vi "Init cDAQ.vi"(8 "error in":errorcluster, 11 "Data in":T1={"Config"={"Hipot"={"COM PORT"=0, "AC to Pack"={"Mode"=0, "Voltage Level"=1000.0, "Low Limit"=0.0, "Hi Limit"=0.001, "ARC Limit"=0.0, "Step"=1.0, "Ramp Time "=0.0, "Test Time "=3.0}, "AC to Pack IR"={"Mode"=0, "Voltage Level IR"=1000.0, "Low Limit"=10000000.0, "Hi Limit"=0.001, "Real Current Limit"=0.0, "Step"=1.0, "Ramp Time "=0.0, "Test Time "=3.0}, "Pack to Case"={"Mode"=0, "Voltage Level"=1000.0, "Low Limit"=10000000.0, "Hi Limit"=0.0, "ARC Limit"=1.0, "Step"=0.0, "Ramp Time "=3.0, "Test Time "=3.0}, "Pack to Case IR"={"Mode"=0, "Voltage Level IR"=1000.0, "Low Limit"=10000000.0, "Hi Limit"=0.0, "Real Current Limit"=0.0, "Step"=1.0, "Ramp Time "=0.0, "Test Time "=3.0}}, "62150H-600 Supply"={"IVI Resource Name"=""}, "6320X E Load Heater"={"IVI Resource Name"=""}, "6320X E Load Compressor"={"IVI Resource Name"=""}, "6320X E Load DCDC"={"IVI Resource Name"=""}, "12061 DMM"={"IVI Resource Name"=""}, "17040 Pack Regen"={"IVI Resource Name"=""}}, "Test Data Ref"=refnum, "Current State Ref"=refnum, "Hipot Ref"=refnum, "Contactors Ref"=refnum, "Equipment Status Ref"=refnum, "TX Packet Info Ref"=refnum, "Pcap Cluster Ref"=refnum, "Eth Adapter ID Ref"=refnum, "Pass/Fail Results Ref"=refnum, "Sequence to Send Ref"=refnum, "Transmit Btn Ref"=refnum, "HW Handles Ref"=refnum, "MPB Status Ref"=refnum, "HVIL Source Ref"=refnum, "HVIL Readback Ref"=refnum, "Coolant Flow Ref"=refnum, "Coolant Temp Ref"=refnum, "Chiller Valve Open % Ref"=refnum} {"Config"."Hipot"."Pack to Case IR"."Test Time" min=0.0 max=999.0 step=0.1 format="%.1f"; "Config"."Hipot"."Pack to Case IR"."Ramp Time" min=0.0 max=999.0 step=0.1 format="%.1f"; "Config"."Hipot"."Pack to Case IR"."Step" min=1.0 max=99.0 step=1.0; "Config"."Hipot"."Pack to Case IR"."Real Current Limit" min=0.0 max=0.03 step=1e-06 format="%.2p"; "Config"."Hipot"."Pack to Case IR"."Voltage Level IR" min=100.0 max=1000.0 step=2.0; "Config"."Hipot"."Pack to Case IR"."Hi Limit" min=0.0 max=50000000000.0 step=10000.0 format="%.2p"; "Config"."Hipot"."Pack to Case IR"."Low Limit" min=100000.0 max=50000000000.0 step=10000.0 format="%.2p"; "Config"."Hipot"."Pack to Case IR"."Mode" items=["AC", "DC", "IR"]; "Config"."Hipot"."Pack to Case"."Test Time" min=0.0 max=999.0 step=0.1 format="%.1f"; "Config"."Hipot"."Pack to Case"."Ramp Time" min=0.0 max=999.0 step=0.1 format="%.1f"; "Config"."Hipot"."Pack to Case"."Step" min=1.0 max=99.0 step=1.0; "Config"."Hipot"."Pack to Case"."ARC Limit" min=0.0 max=0.015 step=1e-06 format="%.2p"; "Config"."Hipot"."Pack to Case"."Hi Limit" min=1e-06 max=0.03 step=1e-06 format="%.2p"; "Config"."Hipot"."Pack to Case"."Low Limit" min=0.0 max=0.03 step=1e-06 format="%.2p"; "Config"."Hipot"."Pack to Case"."Voltage Level" min=100.0 max=6000.0 step=2.0; "Config"."Hipot"."Pack to Case"."Mode" items=["AC", "DC", "IR"]; "Config"."Hipot"."AC to Pack IR"."Test Time" min=0.0 max=999.0 step=0.1 format="%.1f"; "Config"."Hipot"."AC to Pack IR"."Ramp Time" min=0.0 max=999.0 step=0.1 format="%.1f"; "Config"."Hipot"."AC to Pack IR"."Step" min=1.0 max=99.0 step=1.0; "Config"."Hipot"."AC to Pack IR"."Real Current Limit" min=0.0 max=0.03 step=1e-06 format="%.2p"; "Config"."Hipot"."AC to Pack IR"."Voltage Level IR" min=100.0 max=1000.0 step=2.0; "Config"."Hipot"."AC to Pack IR"."Hi Limit" min=0.0 max=50000000000.0 step=10000.0 format="%.2p"; "Config"."Hipot"."AC to Pack IR"."Low Limit" min=100000.0 max=50000000000.0 step=10000.0 format="%.2p"; "Config"."Hipot"."AC to Pack IR"."Mode" items=["AC", "DC", "IR"]; "Config"."Hipot"."AC to Pack"."Test Time" min=0.0 max=999.0 step=0.1 format="%.1f"; "Config"."Hipot"."AC to Pack"."Ramp Time" min=0.0 max=999.0 step=0.1 format="%.1f"; "Config"."Hipot"."AC to Pack"."Step" min=1.0 max=99.0 step=1.0; "Config"."Hipot"."AC to Pack"."ARC Limit" min=0.0 max=0.015 step=1e-06 format="%.2p"; "Config"."Hipot"."AC to Pack"."Hi Limit" min=1e-06 max=0.03 step=1e-06 format="%.2p"; "Config"."Hipot"."AC to Pack"."Low Limit" min=0.0 max=0.03 step=1e-06 format="%.2p"; "Config"."Hipot"."AC to Pack"."Voltage Level" min=100.0 max=6000.0 step=2.0; "Config"."Hipot"."AC to Pack"."Mode" items=["AC", "DC", "IR"]}) -> (0 "error out":errorcluster, 2 "Init cDAQ OK":bool, 3 "Data Out":T1={"Config"={"Hipot"={"COM PORT"=0, "AC to Pack"={"Mode"=0, "Voltage Level"=1000.0, "Low Limit"=0.0, "Hi Limit"=0.001, "ARC Limit"=0.0, "Step"=1.0, "Ramp Time "=0.0, "Test Time "=3.0}, "AC to Pack IR"={"Mode"=0, "Voltage Level IR"=1000.0, "Low Limit"=10000000.0, "Hi Limit"=0.001, "Real Current Limit"=0.0, "Step"=1.0, "Ramp Time "=0.0, "Test Time "=3.0}, "Pack to Case"={"Mode"=0, "Voltage Level"=1000.0, "Low Limit"=10000000.0, "Hi Limit"=0.0, "ARC Limit"=1.0, "Step"=0.0, "Ramp Time "=3.0, "Test Time "=3.0}, "Pack to Case IR"={"Mode"=0, "Voltage Level IR"=1000.0, "Low Limit"=10000000.0, "Hi Limit"=0.0, "Real Current Limit"=0.0, "Step"=1.0, "Ramp Time "=0.0, "Test Time "=3.0}}, "62150H-600 Supply"={"IVI Resource Name"=""}, "6320X E Load Heater"={"IVI Resource Name"=""}, "6320X E Load Compressor"={"IVI Resource Name"=""}, "6320X E Load DCDC"={"IVI Resource Name"=""}, "12061 DMM"={"IVI Resource Name"=""}, "17040 Pack Regen"={"IVI Resource Name"=""}}, "Test Data Ref"=refnum, "Current State Ref"=refnum, "Hipot Ref"=refnum, "Contactors Ref"=refnum, "Equipment Status Ref"=refnum, "TX Packet Info Ref"=refnum, "Pcap Cluster Ref"=refnum, "Eth Adapter ID Ref"=refnum, "Pass/Fail Results Ref"=refnum, "Sequence to Send Ref"=refnum, "Transmit Btn Ref"=refnum, "HW Handles Ref"=refnum, "MPB Status Ref"=refnum, "HVIL Source Ref"=refnum, "HVIL Readback Ref"=refnum, "Coolant Flow Ref"=refnum, "Coolant Temp Ref"=refnum, "Chiller Valve Open % Ref"=refnum} {"Config"."Hipot"."Pack to Case IR"."Test Time" min=0.0 max=999.0 step=0.1 format="%.1f"; "Config"."Hipot"."Pack to Case IR"."Ramp Time" min=0.0 max=999.0 step=0.1 format="%.1f"; "Config"."Hipot"."Pack to Case IR"."Step" min=1.0 max=99.0 step=1.0; "Config"."Hipot"."Pack to Case IR"."Real Current Limit" min=0.0 max=0.03 step=1e-06 format="%.2p"; "Config"."Hipot"."Pack to Case IR"."Voltage Level IR" min=100.0 max=1000.0 step=2.0; "Config"."Hipot"."Pack to Case IR"."Hi Limit" min=0.0 max=50000000000.0 step=10000.0 format="%.2p"; "Config"."Hipot"."Pack to Case IR"."Low Limit" min=100000.0 max=50000000000.0 step=10000.0 format="%.2p"; "Config"."Hipot"."Pack to Case IR"."Mode" items=["AC", "DC", "IR"]; "Config"."Hipot"."Pack to Case"."Test Time" min=0.0 max=999.0 step=0.1 format="%.1f"; "Config"."Hipot"."Pack to Case"."Ramp Time" min=0.0 max=999.0 step=0.1 format="%.1f"; "Config"."Hipot"."Pack to Case"."Step" min=1.0 max=99.0 step=1.0; "Config"."Hipot"."Pack to Case"."ARC Limit" min=0.0 max=0.015 step=1e-06 format="%.2p"; "Config"."Hipot"."Pack to Case"."Hi Limit" min=1e-06 max=0.03 step=1e-06 format="%.2p"; "Config"."Hipot"."Pack to Case"."Low Limit" min=0.0 max=0.03 step=1e-06 format="%.2p"; "Config"."Hipot"."Pack to Case"."Voltage Level" min=100.0 max=6000.0 step=2.0; "Config"."Hipot"."Pack to Case"."Mode" items=["AC", "DC", "IR"]; "Config"."Hipot"."AC to Pack IR"."Test Time" min=0.0 max=999.0 step=0.1 format="%.1f"; "Config"."Hipot"."AC to Pack IR"."Ramp Time" min=0.0 max=999.0 step=0.1 format="%.1f"; "Config"."Hipot"."AC to Pack IR"."Step" min=1.0 max=99.0 step=1.0; "Config"."Hipot"."AC to Pack IR"."Real Current Limit" min=0.0 max=0.03 step=1e-06 format="%.2p"; "Config"."Hipot"."AC to Pack IR"."Voltage Level IR" min=100.0 max=1000.0 step=2.0; "Config"."Hipot"."AC to Pack IR"."Hi Limit" min=0.0 max=50000000000.0 step=10000.0 format="%.2p"; "Config"."Hipot"."AC to Pack IR"."Low Limit" min=100000.0 max=50000000000.0 step=10000.0 format="%.2p"; "Config"."Hipot"."AC to Pack IR"."Mode" items=["AC", "DC", "IR"]; "Config"."Hipot"."AC to Pack"."Test Time" min=0.0 max=999.0 step=0.1 format="%.1f"; "Config"."Hipot"."AC to Pack"."Ramp Time" min=0.0 max=999.0 step=0.1 format="%.1f"; "Config"."Hipot"."AC to Pack"."Step" min=1.0 max=99.0 step=1.0; "Config"."Hipot"."AC to Pack"."ARC Limit" min=0.0 max=0.015 step=1e-06 format="%.2p"; "Config"."Hipot"."AC to Pack"."Hi Limit" min=1e-06 max=0.03 step=1e-06 format="%.2p"; "Config"."Hipot"."AC to Pack"."Low Limit" min=0.0 max=0.03 step=1e-06 format="%.2p"; "Config"."Hipot"."AC to Pack"."Voltage Level" min=100.0 max=6000.0 step=2.0; "Config"."Hipot"."AC to Pack"."Mode" items=["AC", "DC", "IR"]})   [LabVIEW 2020]
uses:
  controls/Data.ctl
  controls/Config.ctl
  controls/Hipot_DC_Config.ctl
  controls/Hipot_IR_Config.ctl
  controls/Test Data Table.ctl
  controls/Hipot.ctl
  controls/Contactors.ctl
  controls/Equipment Status.ctl
  MPB Port Encode Decode/SubVIs/TX Packet Info.ctl
  MPB Port Encode Decode/Ethernet Palette/Controls/VLAN Tag.ctl
  MPB Port Encode Decode/Ethernet Palette/Controls/Pcap Cluster.ctl
  controls/PassFailResults.ctl
  controls/HW Handles.ctl
  controls/MPB Status.ctl
  <vilib>/DAQmx/create/channels.llb/DAQmx Create Channel (AI-Current-Basic).vi
  <vilib>/DAQmx/create/scale.llb/DAQmx Create Scale (Linear).vi
  <vilib>/DAQmx/create/channels.llb/DAQmx Create Channel (DO-Digital Output).vi
  <vilib>/DAQmx/create/channels.llb/DAQmx Create Channel (AO-Current-Basic).vi
  MPB Port Encode Decode/Ethernet Palette.lvlib
panel:
  # "Other"
  # "AC Port Info"
  # "Battery Port Info"
  # "Fault Info"
  # "1"
  # "2"
  # "3"
  # "4"
  # "5"
  # "6"
  # "7"
  # "DC Bus Info"
  # "HAPS Info"
  # "Temps"
  # "1"
  # "2"
  # "Other"
  # "AC Port Info"
  # "Battery Port Info"
  # "Fault Info"
  # "1"
  # "2"
  # "3"
  # "4"
  # "5"
  # "6"
  # "7"
  # "DC Bus Info"
  # "HAPS Info"
  # "Temps"
  # "1"
  # "2"
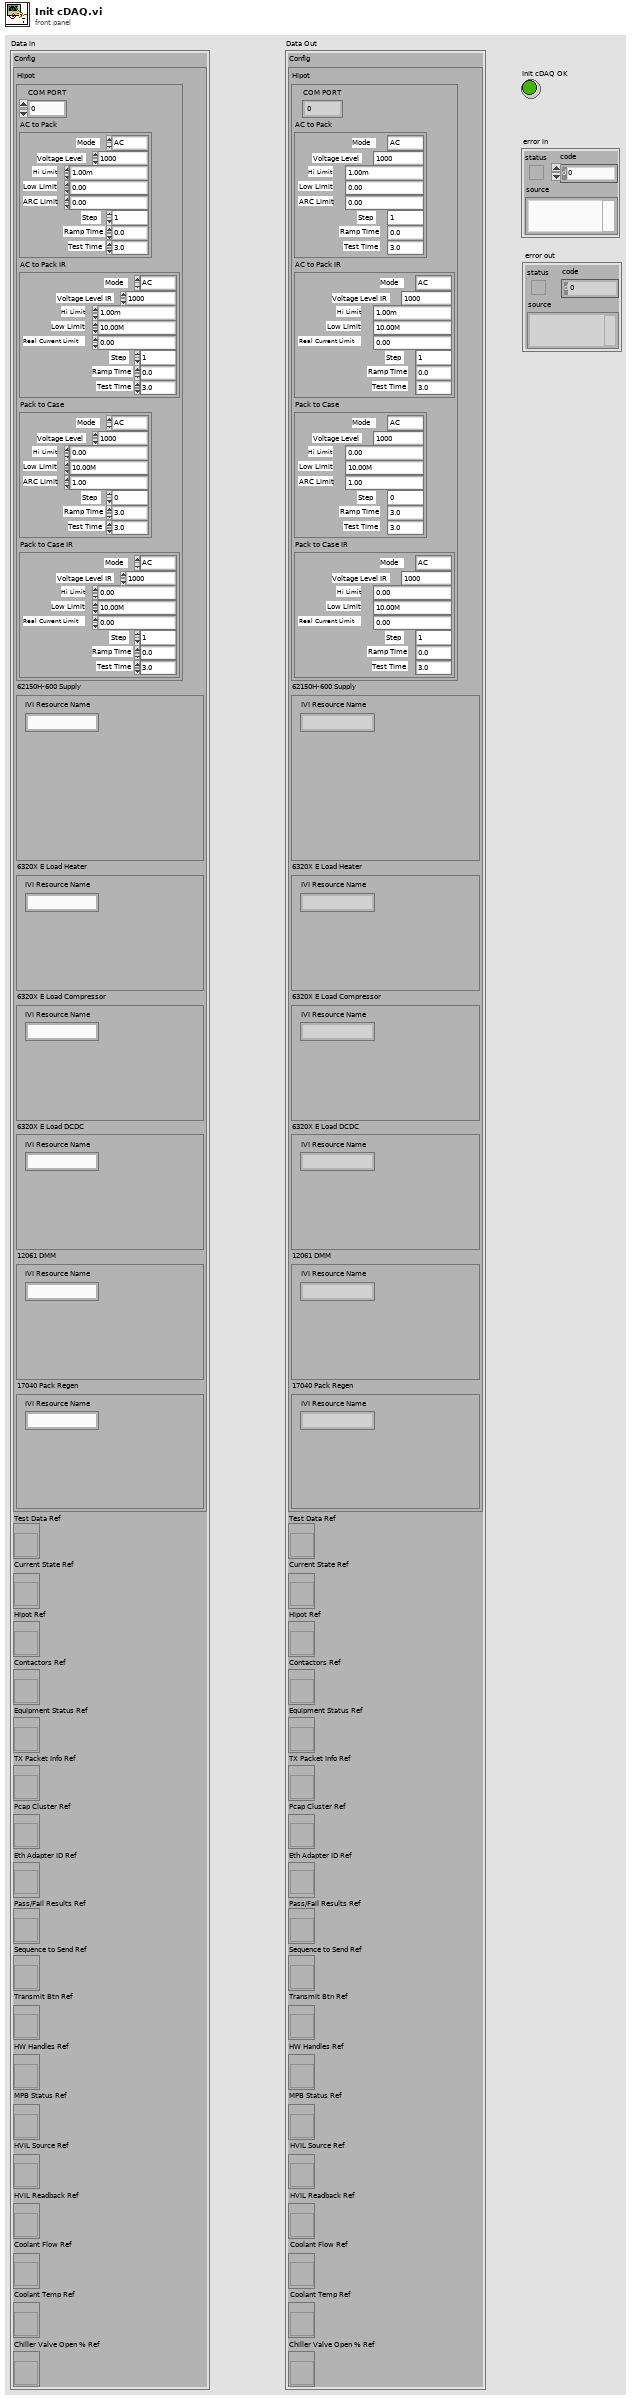
[diagram p1: front panel]
types:
  T1 = typedef "Data.ctl" = cluster{"Config":T2, "Test Data Ref":refnum<vi>, "Current State Ref":refnum<vi>, "Hipot Ref":refnum<vi>, "Contactors Ref":refnum<vi>, "Equipment Status Ref":refnum<vi>, "TX Packet Info Ref":refnum<vi>, "Pcap Cluster Ref":refnum<vi>, "Eth Adapter ID Ref":refnum<vi>, "Pass/Fail Results Ref":refnum<vi>, "Sequence to Send Ref":refnum<vi>, "Transmit Btn Ref":refnum<vi>, "HW Handles Ref":refnum<vi>, "MPB Status Ref":refnum<vi>, "HVIL Source Ref":refnum<vi>, "HVIL Readback Ref":refnum<vi>, "Coolant Flow Ref":refnum<vi>, "Coolant Temp Ref":refnum<vi>, "Chiller Valve Open % Ref":refnum<vi>}
  T2 = typedef "Config.ctl" = cluster{"Hipot":cluster{"COM PORT":u16, "AC to Pack":T3, "AC to Pack IR":T4, "Pack to Case":T3, "Pack to Case IR":T4}, "62150H-600 Supply":cluster{"IVI Resource Name":string}, "6320X E Load Heater":cluster{"IVI Resource Name":string}, "6320X E Load Compressor":cluster{"IVI Resource Name":string}, "6320X E Load DCDC":cluster{"IVI Resource Name":string}, "12061 DMM":cluster{"IVI Resource Name":string}, "17040 Pack Regen":cluster{"IVI Resource Name":string}}
  T3 = typedef "Hipot_DC_Config.ctl" = cluster{"Mode":u16, "Voltage Level":dbl, "Low Limit":dbl, "Hi Limit":dbl, "ARC Limit":dbl, "Step":dbl, "Ramp Time ":dbl, "Test Time ":dbl}
  T4 = typedef "Hipot_IR_Config.ctl" = cluster{"Mode":u16, "Voltage Level IR":dbl, "Low Limit":dbl, "Hi Limit":dbl, "Real Current Limit":dbl, "Step":dbl, "Ramp Time ":dbl, "Test Time ":dbl}
  T5 = typedef "HW Handles.ctl" = cluster{"Hipot Session":refnum<visa-resource-name>, "DC Power Supply Session":refnum<k15>, "E-Load Heater Session":refnum<k15>, "E-Load Compressor Session":refnum<k15>, "E-Load DCDC Session":refnum<k15>, "DMM Session":refnum<k15>, "Pack Regen Session":refnum<k15>, "cDAQ AI Task":refnum<k21>, "cDAQ DO Relay Task":refnum<k21>, "cDAQ DO Contactor Task":refnum<k21>, "cDAQ AO Task":refnum<k21>}
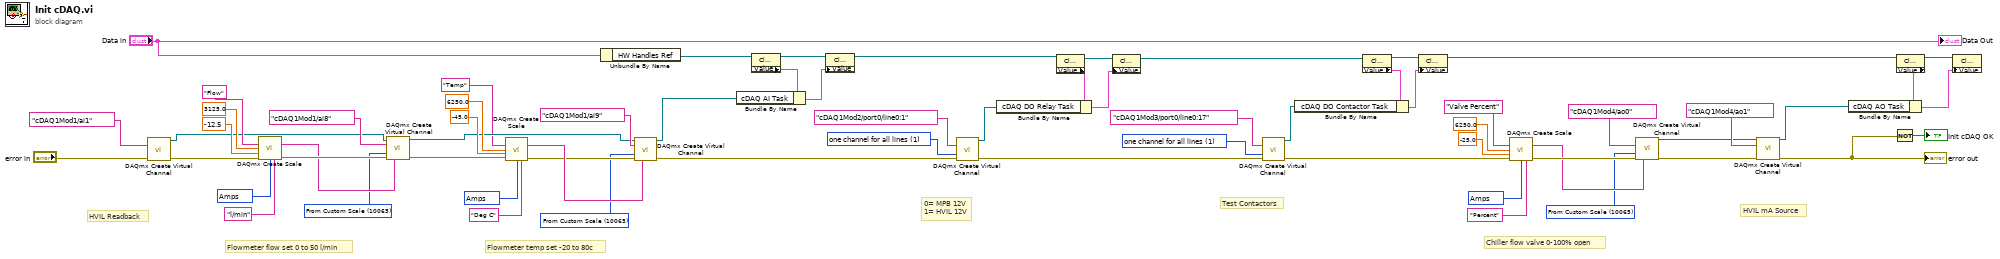
[diagram p0: block diagram]
diagram:
  w1 = 10065 items=["Amps"=10342, "From Custom Scale"=10065] ("units")
  w2 = 10065 items=["Amps"=10342, "From Custom Scale"=10065] ("units")
  w3 = 10065 items=["Amps"=10342, "From Custom Scale"=10065] ("units")
  w34 = 10342 items=["Volts"=10348, "Amps"=10342, "Deg F"=10144, "Deg C"=10143, "Deg R"=10145, "Kelvins"=10325, "Strain"=10299, "Ohms"=10384, "Hz"=10373, "Seconds"=10364, "Meters"=10219, "Inches"=10379, "Degrees"=10146, "Radians"=10273, "Ticks"=10304, "g"=10186, "m/s^2"=12470, "m/s"=15959, "in/s"=15960, "Pascals"=10081, "Newtons"=15875, "Pounds"=15876, "kgf"=15877, "psi"=15879, "bar"=15880, "Nm"=15881, "oz-in"=15882, "lb-in"=15883, "lb-ft"=15884, "Volts/Volt"=15896, "mVolts/Volt"=15897, "pCoulombs"=16103, "Coulombs"=16102, "From TEDS"=12516] ("pre-scaled units")
  w40 = 1 items=["one channel for each line", "one channel for all lines"] ("line grouping")
  w53 = 10342 items=["Volts"=10348, "Amps"=10342, "Deg F"=10144, "Deg C"=10143, "Deg R"=10145, "Kelvins"=10325, "Strain"=10299, "Ohms"=10384, "Hz"=10373, "Seconds"=10364, "Meters"=10219, "Inches"=10379, "Degrees"=10146, "Radians"=10273, "Ticks"=10304, "g"=10186, "m/s^2"=12470, "m/s"=15959, "in/s"=15960, "Pascals"=10081, "Newtons"=15875, "Pounds"=15876, "kgf"=15877, "psi"=15879, "bar"=15880, "Nm"=15881, "oz-in"=15882, "lb-in"=15883, "lb-ft"=15884, "Volts/Volt"=15896, "mVolts/Volt"=15897, "pCoulombs"=16103, "Coulombs"=16102, "From TEDS"=12516] ("pre-scaled units")
  w57 = 10342 items=["Volts"=10348, "Amps"=10342, "Deg F"=10144, "Deg C"=10143, "Deg R"=10145, "Kelvins"=10325, "Strain"=10299, "Ohms"=10384, "Hz"=10373, "Seconds"=10364, "Meters"=10219, "Inches"=10379, "Degrees"=10146, "Radians"=10273, "Ticks"=10304, "g"=10186, "m/s^2"=12470, "m/s"=15959, "in/s"=15960, "Pascals"=10081, "Newtons"=15875, "Pounds"=15876, "kgf"=15877, "psi"=15879, "bar"=15880, "Nm"=15881, "oz-in"=15882, "lb-in"=15883, "lb-ft"=15884, "Volts/Volt"=15896, "mVolts/Volt"=15897, "pCoulombs"=16103, "Coulombs"=16102, "From TEDS"=12516] ("pre-scaled units")
  w66 = 1 items=["one channel for each line", "one channel for all lines"] ("line grouping")
  # "HVIL Readback"
  # "Test Contactors"
  # "0= MPB 12V\n1= HVIL 12V"
  # "HVIL mA Source"
  # "Chiller flow valve 0-100% open"
  # "Flowmeter temp set -20 to 80c"
  # "Flowmeter flow set 0 to 50 l/min"
  n1 = call-poly <vilib>:"DAQmx Create Virtual Channel.vi"("physical channels"=tag "cDAQ1Mod1/ai1", "error in"="error in") -> ("task out"=w42:refnum<k21>, "error out"=w43:errorcluster)  [unwired: 12 in]
  n2 = call-poly <vilib>:"DAQmx Create Scale.vi"("name"="Flow", "slope"=3125.0, "y-intercept"=-12.5, "error in"=w43, "pre-scaled units"=w57, "scaled units"="l/min") -> ("scale out"=w54:tag, "error out"=w55:errorcluster)  [unwired: 8 in]
  n3 = call-poly <vilib>:"DAQmx Create Virtual Channel.vi"("task in"=w42, "physical channels"=tag "cDAQ1Mod1/ai8", "units"=w3, "error in"=w55, "custom scale name"=w54) -> ("task out"=w49:refnum<k21>, "error out"=w48:errorcluster)  [unwired: 9 in]
  n4 = call-poly <vilib>:"DAQmx Create Scale.vi"("name"="Temp", "slope"=6250.0, "y-intercept"=-45.0, "error in"=w48, "pre-scaled units"=w53, "scaled units"="Deg C") -> ("scale out"=w47:tag, "error out"=w46:errorcluster)  [unwired: 8 in]
  n5 = Unbundle By Name("Data in") -> ("HW Handles Ref"=w22:refnum<vi>)
  n6 = call-poly <vilib>:"DAQmx Create Virtual Channel.vi"("task in"=w49, "physical channels"=tag "cDAQ1Mod1/ai9", "units"=w2, "error in"=w46, "custom scale name"=w47) -> ("task out"=w6:refnum<k21>, "error out"=w7:errorcluster)  [unwired: 9 in]
  n7 = property class="Clust (strict)"(reference=w22) -> (reference out=w24:refnum<vi>, "Value"=w25:T5)  [unwired: 1 in, 1 out]
  n8 = Bundle By Name(cluster=w25, "cDAQ AI Task"=w6) -> (w23:T5)
  n9 = property class="Clust (strict)"(reference=w24, "Value"=w23) -> (reference out=w19:refnum<vi>)  [unwired: 1 in, 1 out]
  n10 = call-poly <vilib>:"DAQmx Create Virtual Channel.vi"("lines"=tag "cDAQ1Mod2/port0/line0:1", "line grouping"=w40, "error in"=w7) -> ("task out"=w17:refnum<k21>, "error out"=w39:errorcluster)  [unwired: 11 in]
  n11 = property class="Clust (strict)"(reference=w19) -> (reference out=w18:refnum<vi>, "Value"=w20:T5)  [unwired: 1 in, 1 out]
  n12 = Bundle By Name(cluster=w20, "cDAQ DO Relay Task"=w17) -> (w21:T5)
  n13 = property class="Clust (strict)"(reference=w18, "Value"=w21) -> (reference out=w13:refnum<vi>)  [unwired: 1 in, 1 out]
  n14 = call-poly <vilib>:"DAQmx Create Virtual Channel.vi"("lines"=tag "cDAQ1Mod3/port0/line0:17" ("physical channels"), "line grouping"=w66, "error in"=w39) -> ("task out"=w12:refnum<k21>, "error out"=w30:errorcluster)  [unwired: 11 in]
  n15 = property class="Clust (strict)"(reference=w13) -> (reference out=w16:refnum<vi>, "Value"=w15:T5)  [unwired: 1 in, 1 out]
  n16 = Bundle By Name(cluster=w15, "cDAQ DO Contactor Task"=w12) -> (w14:T5)
  n17 = property class="Clust (strict)"(reference=w16, "Value"=w14) -> (reference out=w9:refnum<vi>)  [unwired: 1 in, 1 out]
  n18 = call-poly <vilib>:"DAQmx Create Scale.vi"("name"="Valve Percent", "slope"=6250.0, "y-intercept"=-25.0, "error in"=w30, "pre-scaled units"=w34, "scaled units"="Percent") -> ("scale out"=w35:tag, "error out"=w37:errorcluster)  [unwired: 8 in]
  n19 = call-poly <vilib>:"DAQmx Create Virtual Channel.vi"("physical channels"=tag "cDAQ1Mod4/ao0", "units"=w1, "error in"=w37, "custom scale name"=w35) -> ("task out"=w27:refnum<k21>, "error out"=w28:errorcluster)  [unwired: 10 in]
  n20 = call-poly <vilib>:"DAQmx Create Virtual Channel.vi"("task in"=w27, "physical channels"=tag "cDAQ1Mod4/ao1", "error in"=w28) -> ("task out"=w4:refnum<k21>, "error out"=w5:errorcluster)  [unwired: 11 in]
  "error out" <- w5
  n21 = Not(x=w5) -> (.not. x?=→"Init cDAQ OK":bool)
  n22 = property class="Clust (strict)"(reference=w9) -> (reference out=w8:refnum<vi>, "Value"=w10:T5)  [unwired: 1 in, 1 out]
  n23 = Bundle By Name(cluster=w10, "cDAQ AO Task"=w4) -> (w11:T5)
  n24 = property class="Clust (strict)"(reference=w8, "Value"=w11) -> ()  [unwired: 1 in, 2 out]
  "Data Out" <- "Data in"
